vi "Read Required Signals.vi"(8 "error in (no error)":errorcluster, 11 "Instruments in":refnum<class "Instruments.lvclass">) -> (0 "error out":errorcluster, 2 "Required Signals":string[](array[string]), 3 "Instruments out":refnum<class "Instruments.lvclass">)   [LabVIEW 2023, in "Instruments.lvlib" / "Instruments.lvclass"]
doc: "This override routine is used to create default signals to be loaded in to the signal list. \nThis is a placeholder routine for editor functions in later development.\n\n<b>Instrument</b> - There is no implementation at the instrument layer, this is provided as a pass through."
uses:
  Library/Instruments.lvclass
  builds/Framework/Configuration.lvlibp/Library/Configuration.lvclass
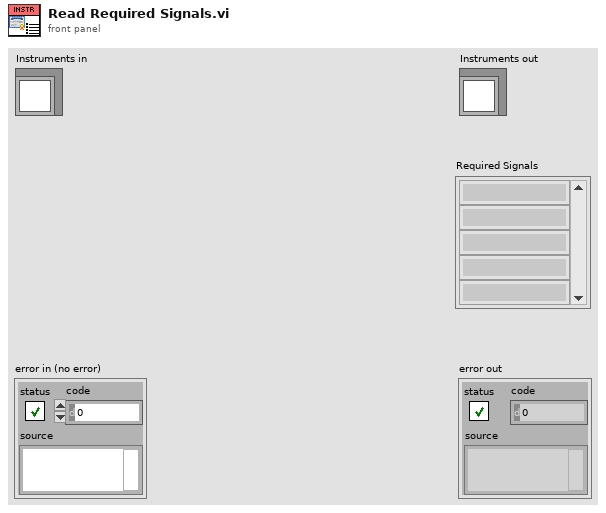
[diagram p1: front panel]
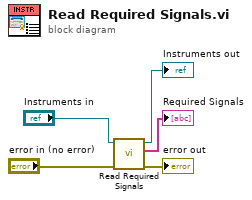
[diagram p0: block diagram]
diagram:
  n1 = call-parent "Read Required Signals.vi"("error in (no error)"="error in (no error)", "Configuration in"="Instruments in") -> ("error out"=→"error out":errorcluster, "Required Signals"=→"Required Signals":string[], "Configuration out"=→"Instruments out":refnum<class "Instruments.lvclass">)  [unwired: 7 in]
